vi "GlobalInitializeFlag.vi"() -> ()   [LabVIEW 2010]
panel:
  in  "Camera Initialized":u32
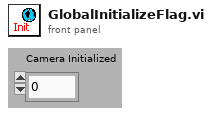
[diagram p1: front panel]
diagram:
